vi "Save MATLAB Results.vi"(9 "NumValues":dbl[][](array[numeric])=[[1.0, 200.0, 0.0, 1.2], [3.0, 200.0, 0.0, 1.3], [4.0, 200.0, 0.0, 1.4]], 10 "NumNames":string[](array[string])=["Theta", "X", "Y", "U"]) -> ()   [LabVIEW 2022 SP3]
panel:
  in  "TimetraceNames":string[](array[string])=["Theta", "X", "Y", "U"]
  in  "TimetraceValues":dbl[][](array[numeric])=[[1.0, 200.0, 0.0, 1.2], [3.0, 200.0, 0.0, 1.3], [4.0, 200.0, 0.0, 1.4]]
  in  "Path":path
  in  "Filename":string="check7.mat"
  in  "String Names":string[](array[string])=["Filename", "User", "Date", "Day"]
  in  "String Array":string[][](array[string])=[["file1", "Paul", "23/5/24", "Mon"], ["file1", "Paul", "24/5/24", "Tues"], ["file1", "Paul", "25/5/24", "Wed"]]
  out "N":dbl
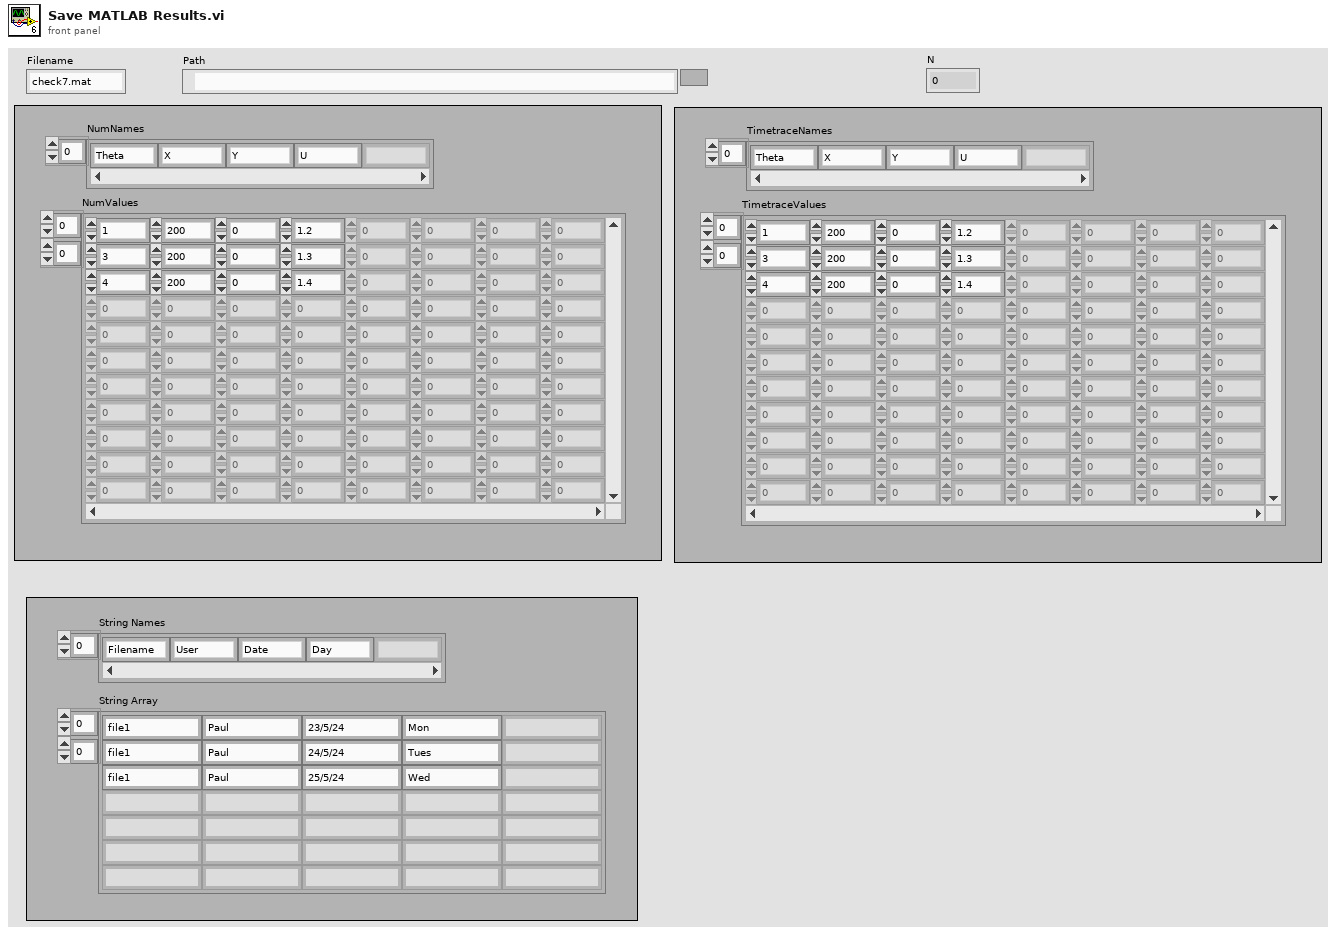
[diagram p1: front panel]
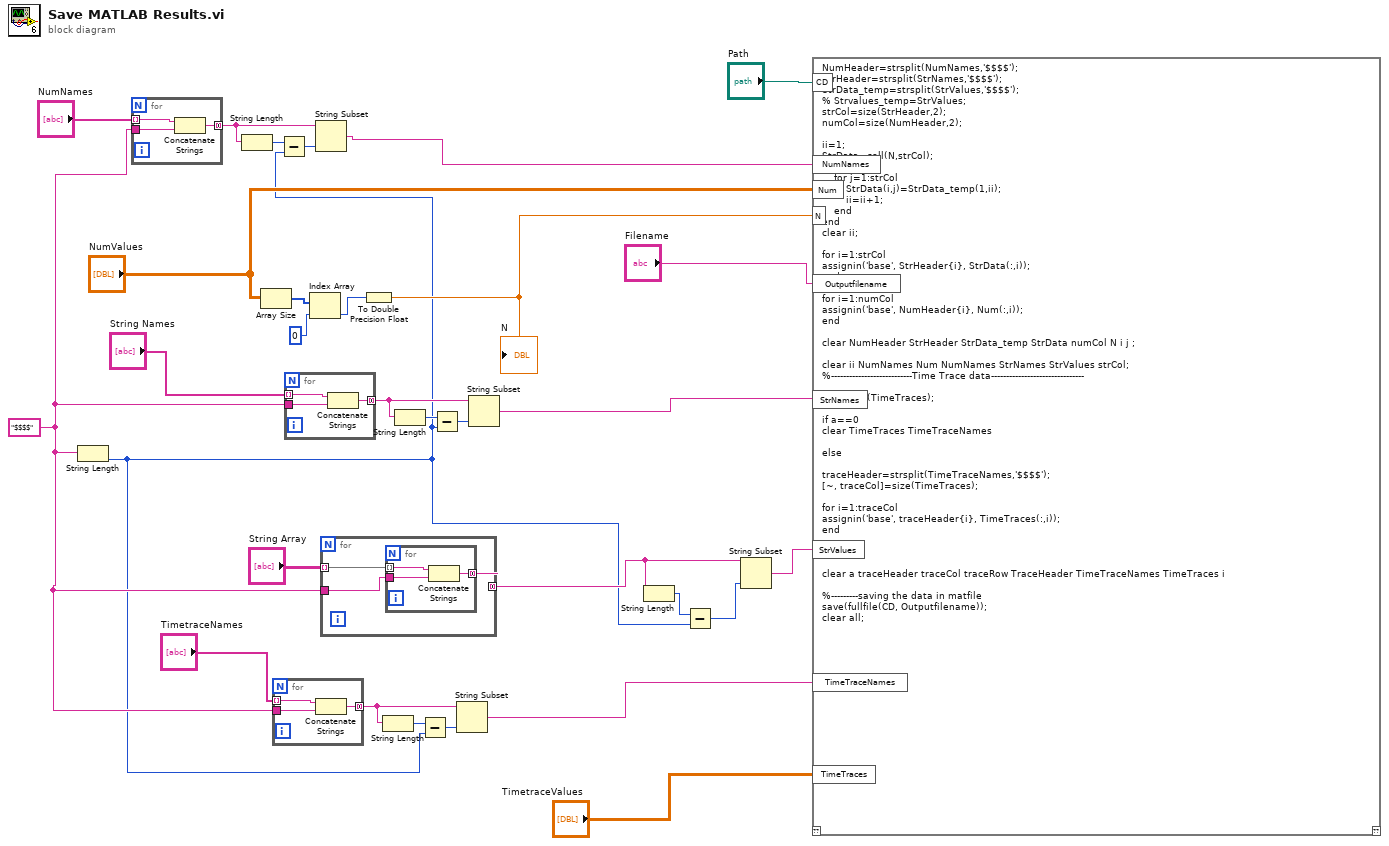
[diagram p0: block diagram]
diagram:
  w4 = "$$$$" ("string")
  n1 = String Length(string=w4) -> (length=w3:i32)
  n2 = for {
    tunnel: "NumNames" -> [w33] mode=indexing
    tunnel: [w32] -> w28 mode=concatenating
    tunnel: w4 -> [w31]
    n3 = Concatenate Strings(w33, w31) -> (w32:string)
  }
  n4 = String Length(string=w28) -> (length=w29:i32)
  n5 = Array Size(array="NumValues") -> (size(s)=w24:i32[])
  n6 = for {
    tunnel: "TimetraceNames" -> [w36] mode=indexing
    tunnel: [w35] -> w7 mode=concatenating
    tunnel: w4 -> [w34]
    n7 = Concatenate Strings(w36, w34) -> (w35:string)
  }
  n8 = Subtract(x=w29, y=w3) -> (x-y=w27:i32)
  n9 = for {
    tunnel: "String Names" -> [w39] mode=indexing
    tunnel: [w38] -> w19 mode=concatenating
    tunnel: w4 -> [w37]
    n10 = Concatenate Strings(w39, w37) -> (w38:string)
  }
  n11 = Index Array(array=w24, index=0) -> (element=w23:i32)
  n12 = String Subset(string=w28, length (rest)=w27) -> (substring=w26:string)  [unwired: 1 in]
  n13 = for {
    tunnel: "String Array" -> [w42] mode=indexing
    tunnel: [w41] -> w12 mode=concatenating
    tunnel: w4 -> [w40]
    n14 = for {
      tunnel: w42 -> [w45] mode=indexing
      tunnel: [w44] -> w41 mode=concatenating
      tunnel: w40 -> [w43]
      n15 = Concatenate Strings(w45, w43) -> (w44:string)
    }
  }
  n16 = To Double Precision Float(number=w23) -> (double precision float=w21:dbl)
  "N" <- w21
  n17 = String Length(string=w7) -> (length=w8:i32)
  n18 = String Length(string=w19) -> (length=w18:i32)
  n19 = Subtract(x=w8, y=w3) -> (x-y=w6:i32)
  n20 = Subtract(x=w18, y=w3) -> (x-y=w20:i32)
  n21 = String Subset(string=w7, length (rest)=w6) -> (substring=w2:string)  [unwired: 1 in]
  n22 = String Subset(string=w19, length (rest)=w20) -> (substring=w15:string)  [unwired: 1 in]
  n23 = String Length(string=w12) -> (length=w14:i32)
  n24 = Subtract(x=w14, y=w3) -> (x-y=w13:i32)
  n25 = String Subset(string=w12, length (rest)=w13) -> (substring=w11:string)  [unwired: 1 in]
  n26 = script code="NumHeader=strsplit(NumNames,'$$$$');\nStrHeader=strsplit(StrNames,'$$$$');\nStrData_temp=strsplit(StrValues,'$$$$');\n% Strvalues_temp=StrValues;\nstrCol=size(StrHeader,2);\nnumCol=size(NumHeader,2);\n\nii=1;\nStrData=cell(N,strCol);\nfor i=1:N\n    for j=1:strCol\n        StrData(i,j)=StrData_temp(1,ii);\n        ii=ii+1;\n    end\nend\nclear ii;\n\nfor i=1:strCol\nassignin('base', StrHeader{i}, StrData(:,i));\nend\n\nfor i=1:numCol\nassignin('base', NumHeader{i}, Num(:,i));\nend\n\nclear NumHeader StrHeader StrData_temp StrData numCol N i j ;\n\nclear ii NumNames Num NumNames StrNames StrValues strCol;\n%---------------------------Time Trace data-------------------------------\n\na=length(TimeTraces);\n\nif a==0\nclear TimeTraces TimeTraceNames\n\nelse\n\ntraceHeader=strsplit(TimeTraceNames,'$$$$');\n[~, traceCol]=size(TimeTraces);\n\nfor i=1:traceCol\nassignin('base', traceHeader{i}, TimeTraces(:,i));\nend\n\nend\n\nclear a traceHeader traceCol traceRow TraceHeader TimeTraceNames TimeTraces i\n\n%---------saving the data in matfile\nsave(fullfile(CD, Outputfilename));\nclear all;"("Num"="NumValues", "CD"="Path", "NumNames"=w26, "StrValues"=w11, "N"=w21, "StrNames"=w15, "Outputfilename"="Filename", "TimeTraceNames"=w2, "TimeTraces"="TimetraceValues") -> ()  [unwired: 1 in, 1 out]
